vi "ZeroMQ_FOC.vi"() -> ()   [LabVIEW 2018]
uses:
  <vilib>/addons/zeromq/socket_type.ctl
  <vilib>/addons/zeromq/socket_options.ctl
  <vilib>/addons/zeromq/zeromq.lvlib
  <vilib>/addons/zeromq/zmq_socket.lvclass
  <vilib>/addons/zeromq/zmq_context.lvclass
panel:
  out "command":string
  in  "stop 3":bool
  out "error out 3":errorcluster
  out "error out 2":errorcluster
  out "message":string
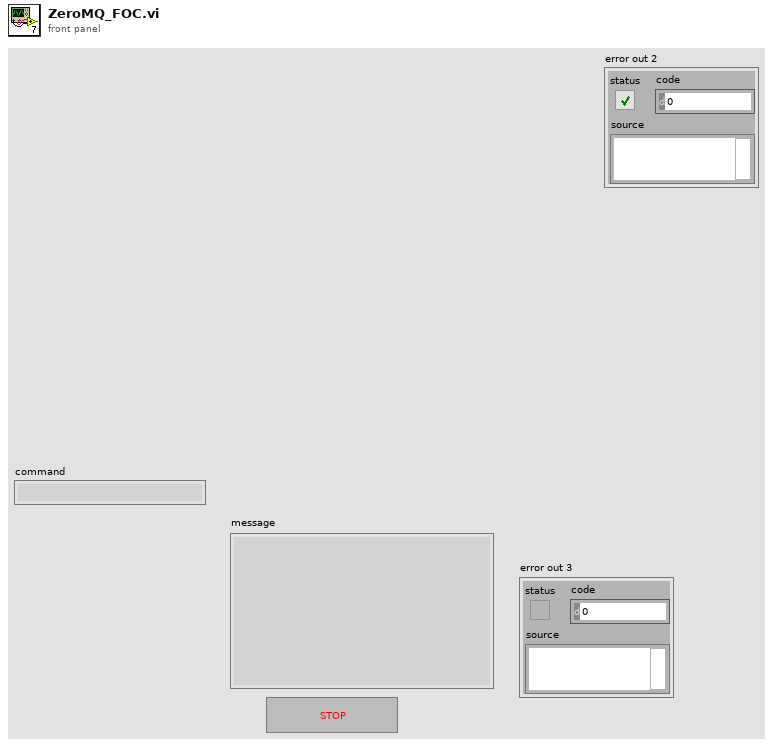
[diagram p1: front panel]
types:
  T1 = cluster{"ID":u32, "Address":string, "Service Name 1":string, "Service Name 2":string, "queue TX":refnum<queue>, "queue RX":refnum<queue>, "Port 1":u32, "Port 2":u32}
  T2 = typedef "zeromq.lvlib/socket_type.ctl" = enum8{"ZMQ_PAIR", "ZMQ_PUB", "ZMQ_SUB", "ZMQ_REQ", "ZMQ_REP", "ZMQ_DEALER", "ZMQ_ROUTER", "ZMQ_PULL", "ZMQ_PUSH", "ZMQ_XPUB", "ZMQ_XSUB", "ZMQ_STREAM", "ZMQ_SERVER", "ZMQ_CLIENT", "ZMQ_RADIO", "ZMQ_DISH", "ZMQ_GATHER", "ZMQ_SCATTER", "ZMQ_DGRAM"}
  T3 = typedef "zeromq.lvlib/socket_options.ctl" = enum8{"NONE", "ZMQ_HWM", "<2>", "ZMQ_SWAP", "ZMQ_AFFINITY", "ZMQ_ROUTING_ID", "ZMQ_SUBSCRIBE", "ZMQ_UNSUBSCRIBE", "ZMQ_RATE", "ZMQ_RECOVERY_IVL", "ZMQ_MCAST_LOOP", "ZMQ_SNDBUF", "ZMQ_RCVBUF", "ZMQ_RCVMORE", "ZMQ_FD", "ZMQ_EVENTS", "ZMQ_TYPE", "ZMQ_LINGER", "ZMQ_RECONNECT_IVL", "ZMQ_BACKLOG", "ZMQ_RECOVERY_IVL_MSEC", "ZMQ_RECONNECT_IVL_MAX", "ZMQ_MAXMSGSIZE", "ZMQ_SNDHWM", "ZMQ_RCVHWM", "ZMQ_MULTICAST_HOPS", "<26>", "ZMQ_RCVTIMEO", "ZMQ_SNDTIMEO", "<29>", "<30>", "ZMQ_IPV4ONLY", "ZMQ_LAST_ENDPOINT", "ZMQ_ROUTER_MANDATORY", "ZMQ_TCP_KEEPALIVE", "ZMQ_TCP_KEEPALIVE_CNT", "ZMQ_TCP_KEEPALIVE_IDLE", "ZMQ_TCP_KEEPALIVE_INTVL", "ZMQ_TCP_ACCEPT_FILTER", "ZMQ_IMMEDIATE", "ZMQ_XPUB_VERBOSE", "ZMQ_ROUTER_RAW", "ZMQ_IPV6", "ZMQ_MECHANISM", "ZMQ_PLAIN_SERVER", "ZMQ_PLAIN_USERNAME", "ZMQ_PLAIN_PASSWORD", "ZMQ_CURVE_SERVER", "ZMQ_CURVE_PUBLICKEY", "ZMQ_CURVE_SECRETKEY", "ZMQ_CURVE_SERVERKEY", "ZMQ_PROBE_ROUTER", "ZMQ_REQ_CORRELATE", "ZMQ_REQ_RELAXED", "ZMQ_CONFLATE", "ZMQ_ZAP_DOMAIN", "ZMQ_ROUTER_HANDOVER", "ZMQ_TOS", "ZMQ_IPC_FILTER_PID", "ZMQ_IPC_FILTER_UID", "ZMQ_IPC_FILTER_GID", "ZMQ_CONNECT_ROUTING_ID", "ZMQ_GSSAPI_SERVER", "ZMQ_GSSAPI_PRINCIPAL", "ZMQ_GSSAPI_SERVICE_PRINCIPAL", "ZMQ_GSSAPI_PLAINTEXT", "ZMQ_HANDSHAKE_IVL", "<67>", "ZMQ_SOCKS_PROXY", "ZMQ_XPUB_NODROP", "ZMQ_BLOCKY", "ZMQ_XPUB_MANUAL", "ZMQ_XPUB_WELCOME_MSG", "ZMQ_STREAM_NOTIFY", "ZMQ_INVERT_MATCHING", "ZMQ_HEARTBEAT_IVL", "ZMQ_HEARTBEAT_TTL", "ZMQ_HEARTBEAT_TIMEOUT", "ZMQ_XPUB_VERBOSER", "ZMQ_CONNECT_TIMEOUT", "ZMQ_TCP_MAXRT", "ZMQ_THREAD_SAFE", "<82>", "<83>", "ZMQ_MULTICAST_MAXTPDU", "ZMQ_VMCI_BUFFER_SIZE", "ZMQ_VMCI_BUFFER_MIN_SIZE", "ZMQ_VMCI_BUFFER_MAX_SIZE", "ZMQ_VMCI_CONNECT_TIMEOUT", "ZMQ_USE_FD", "ZMQ_GSSAPI_PRINCIPAL_NAMETYPE", "ZMQ_GSSAPI_SERVICE_PRINCIPAL_NAMETYPE", "ZMQ_BINDTODEVICE", "ZMQ_ZAP_ENFORCE_DOMAIN", "ZMQ_LOOPBACK_FASTPATH", "ZMQ_METADATA", "ZMQ_MULTICAST_LOOP", "ZMQ_ROUTER_NOTIFY"}
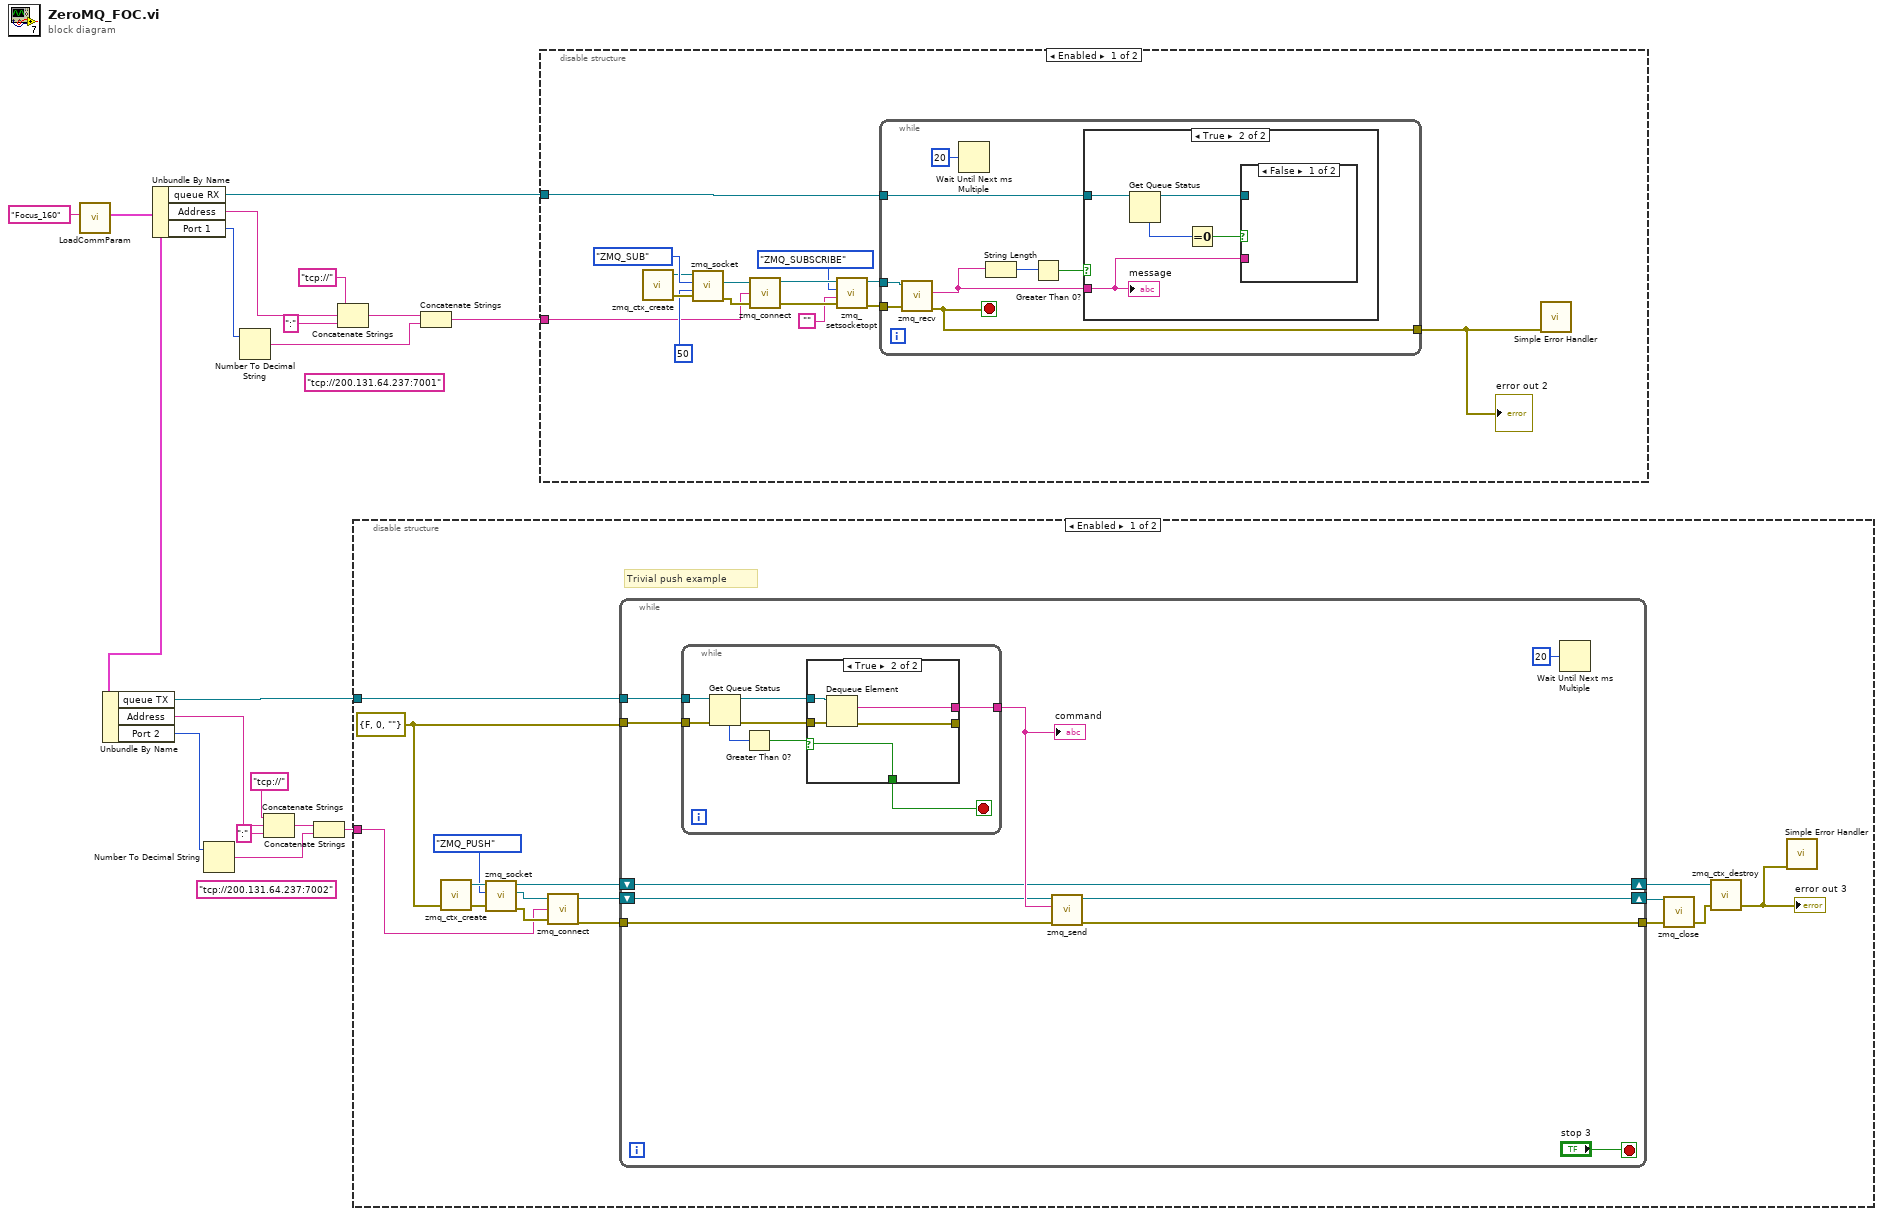
[diagram p0: block diagram]
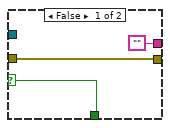
[diagram p2: hidden frame]
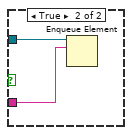
[diagram p5: hidden frame]
diagram:
  (unwired) "tcp://200.131.64.237:7002" ("endpoint")
  (unwired) "tcp://200.131.64.237:7001" ("endpoint")
  n1 = call "LoadCommParam.vi"("section name"="Focus_160") -> ("output cluster"=w1:T1)  [unwired: 10 in]
  n2 = Unbundle By Name(w1) -> ("queue TX"=w10:refnum<queue>, "Address"=w5:string, "Port 2"=w4:u32)
  n3 = Unbundle By Name(w1) -> ("queue RX"=w2:refnum<queue>, "Address"=w17:string, "Port 1"=w16:u32)
  n4 = Number To Decimal String(number=w4) -> (decimal integer string=w9:string)  [unwired: 1 in]
  n5 = Number To Decimal String(number=w16) -> (decimal integer string=w15:string)  [unwired: 1 in]
  n6 = Concatenate Strings("tcp://" ("string"), w5, ":" ("string")) -> (w8:string)
  n7 = Concatenate Strings(w8, w9) -> (w3:string)
  n8 = Concatenate Strings("tcp://" ("string"), w17, ":" ("string")) -> (w14:string)
  n9 = disable-structure shown="Enabled" {
    disable-tunnel: w10 -> [w34 _]
    disable-tunnel: w3 -> [w22 _]
    frame Enabled {
      w25 = errorcluster {"status"=FALSE, "code"=0, "source"=""} ("error out")
      # "Trivial push example"
      n10 = call <vilib>:"zmq_ctx_create.vi"("error in"=w25) -> ("error out"=w30:errorcluster, "context out"=w29:refnum<class "zmq_context.lvclass">)  [unwired: 3 in]
      n11 = call <vilib>:"zmq_socket.vi"("error in"=w30, "socket type"=socket_type."ZMQ_PUSH", "context in"=w29) -> ("error out"=w23:errorcluster, "socket out"=w24:refnum<class "zmq_socket.lvclass">, "context out"=w19:refnum<class "zmq_context.lvclass">)  [unwired: 2 in]
      n12 = call <vilib>:"zmq_connect.vi"("error in"=w23, "endpoint"=w22, "socket in"=w24) -> ("error out"=w21:errorcluster, "socket out"=w20:refnum<class "zmq_socket.lvclass">)  [unwired: 1 in]
      n13 = while {
        tunnel: w34 -> [w44]
        tunnel: w25 -> [w41]
        tunnel: [w39] -> w32
        tunnel: w21 -> [w37]
        shift-right: [w35] -> w27
        shift-left: w19 -> [w35]
        shift-right: [w38] -> w31
        shift-left: w20 -> [w36]
        stop <- "stop 3" stop-if-true
        n14 = while {
          tunnel: w44 -> [w51]
          tunnel: w41 -> [w50]
          tunnel: [w46] -> w43
          stop <- w45 stop-if-true
          n15 = Get Queue Status(queue=w51, error in (no error)=w50) -> (queue out=w47:refnum<queue>, error out=w48:errorcluster, # elements in queue=w52:i32)  [unwired: 1 in, 5 out]
          n16 = Greater Than 0?(x=w52) -> (x > 0?=w49:bool)
          n17 = case shown="True" w49 {
            selector: w49 -> [w53 w56]
            tunnel: w48 -> [w55 w60]
            tunnel: w47 -> [_ w59]
            tunnel: [w55 w58] -> _
            tunnel: ["" w57] -> w46
            tunnel: [w53 w56] -> w45
            frame False {
            }
            frame True {
              n18 = Dequeue Element(queue=w59, error in (no error)=w60) -> (element=w57:string, error out=w58:errorcluster)  [unwired: 1 in, 2 out]
            }
          }
        }
        "command" <- w43
        n19 = call <vilib>:"zmq_send.vi"("error in"=w37, "data"=w43, "socket in"=w36) -> ("error out"=w39:errorcluster, "socket out"=w38:refnum<class "zmq_socket.lvclass">)  [unwired: 4 in]
        n20 = Wait Until Next ms Multiple(millisecond multiple=u32 20) -> ()  [unwired: 1 out]
      }
      n21 = call <vilib>:"zmq_close.vi"("error in"=w32, "socket"=w31) -> ("error out"=w33:errorcluster)  [unwired: 3 in]
      n22 = call <vilib>:"zmq_ctx_destroy.vi"("error in"=w33, "context in"=w27) -> ("error out"=w26:errorcluster)  [unwired: 3 in]
      "error out 3" <- w26
      n23 = call <vilib>:"Simple Error Handler.vi"("error in (no error)"=w26) -> ()  [unwired: 4 in, 5 out]
    }
    frame Disabled {
    }
  }
  n24 = Concatenate Strings(w14, w15) -> (w11:string)
  n25 = disable-structure shown="Enabled" {
    disable-tunnel: w2 -> [w62 _]
    disable-tunnel: w11 -> [w61 _]
    frame Enabled {
      n26 = call <vilib>:"zmq_ctx_create.vi"() -> ("error out"=w74:errorcluster, "context out"=w64:refnum<class "zmq_context.lvclass">)  [unwired: 4 in]
      n27 = call <vilib>:"zmq_socket.vi"("error in"=w74, "linger (ms)"=50, "socket type"=socket_type."ZMQ_SUB", "context in"=w64) -> ("error out"=w73:errorcluster, "socket out"=w65:refnum<class "zmq_socket.lvclass">)  [unwired: 1 in, 1 out]
      n28 = call <vilib>:"zmq_connect.vi"("error in"=w73, "endpoint"=w61, "socket in"=w65) -> ("error out"=w71:errorcluster, "socket out"=w72:refnum<class "zmq_socket.lvclass">)  [unwired: 1 in]
      n29 = call <vilib>:"zmq_setsocketopt.vi"("error in"=w71, "value"="", "option"=socket_options."ZMQ_SUBSCRIBE", "socket in"=w72) -> ("error out"=w70:errorcluster, "socket out"=w69:refnum<class "zmq_socket.lvclass">)  [unwired: 2 in]
      n30 = while {
        tunnel: w69 -> [w81]
        tunnel: w70 -> [w83]
        tunnel: [w82] -> w66
        tunnel: w62 -> [w78]
        stop <- w82 stop-if-true
        n31 = call <vilib>:"zmq_recv.vi"("error in"=w83, "socket in"=w81) -> ("error out"=w82:errorcluster, "data"=w77:string)  [unwired: 3 in, 3 out]
        n32 = Wait Until Next ms Multiple(millisecond multiple=u32 20) -> ()  [unwired: 1 out]
        n33 = String Length(string=w77) -> (length=w80:i32)
        n34 = Greater Than 0?(x=w80) -> (x > 0?=w79:bool)
        n35 = case shown="True" w79 {
          tunnel: w78 -> [_ w87]
          tunnel: w77 -> [_ w84]
          frame False {
          }
          frame True {
            n36 = Get Queue Status(queue=w87) -> (queue out=w85:refnum<queue>, # elements in queue=w88:i32)  [unwired: 2 in, 6 out]
            n37 = Equal To 0?(x=w88) -> (x = 0?=w86:bool)
            n38 = case shown="False" w86 {
              tunnel: w85 -> [_ w90]
              tunnel: w84 -> [_ w89]
              frame False {
              }
              frame True {
                n39 = Enqueue Element(queue=w90, element=w89) -> ()  [unwired: 2 in, 3 out]
              }
            }
            "message" <- w84
          }
        }
      }
      "error out 2" <- w66
      n40 = call <vilib>:"Simple Error Handler.vi"("error in (no error)"=w66) -> ()  [unwired: 4 in, 5 out]
    }
    frame Disabled {
    }
  }
